vi "Result.Attributes plus Numeric into Results Table.vi"(6 "Meas":T1[](array[typedef]) {"Status" items=["LOG", "PASS", "FAIL", "ERROR"]}, 7 "File Data Objs":T3[](array[typedef]), 8 "Show Only Failures":bool, 9 "Filter":string, 10 "Attribute Data":T7[](array[typedef]) {"Status" items=["LOG", "PASS", "FAIL", "ERROR"]}, 11 "Numeric Data":T5[](array[typedef]) {"Status" items=["LOG", "PASS", "FAIL", "ERROR"]}) -> (1 "Failing":bool, 3 "Results Table":T4[](array[typedef]))   [LabVIEW 2024]
uses:
  Result.Attribute.ctl
  Result.Measurement and Attribute Item Status.ctl
  Result.Numeric.ctl
  Result.Limit Type.ctl
  Result.Results Table Record.ctl
  Reports/Report.Result FileDataObject.ctl
  Result.Measurement Item.ctl
  <vilib>/Utility/error.llb/Trim Whitespace One-Sided.vi
panel:
  in  "N/A Filler":string="n/a"
  in  "Precision (3)":i16=3
  # "Step                          Name                                             Value                      Units    LimType       LL           UL          Result        Code                     Description"
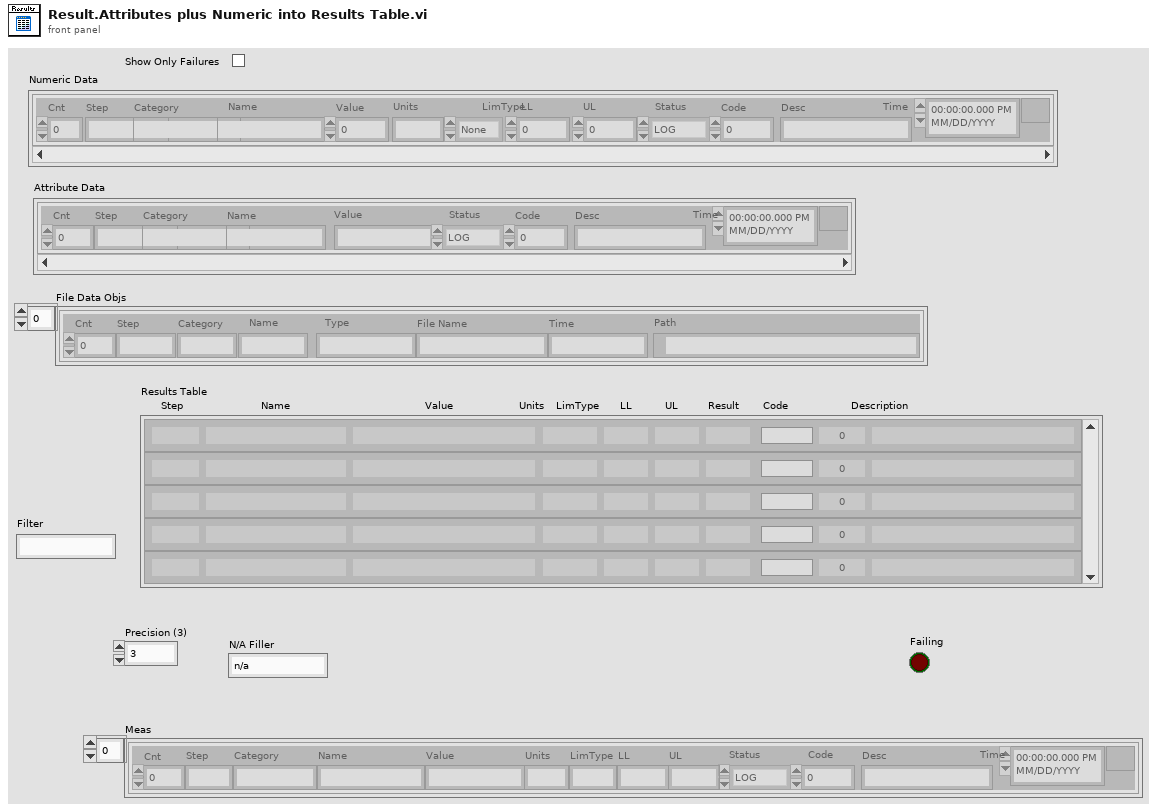
[diagram p1: front panel]
types:
  T1 = typedef "Result.Measurement Item.ctl" = cluster{"Cnt":i32, "Step":string, "Category":string, "Name":string, "Value":string, "Units":string, "LimType":string, "LL":string, "UL":string, "Status":T2, "Code":i32, "Desc":string, "Time":timestamp}
  T2 = typedef "Result.Measurement and Attribute Item Status.ctl" = i32
  T3 = typedef "Report.Result FileDataObject.ctl" = cluster{"Cnt":i32, "Step":string, "Category":string, "Name":string, "Type":string, "File Name":string, "Time":string, "Path":path}
  T4 = typedef "Result.Results Table Record.ctl" = cluster{"Cnt":i32, "Step":string, "Category":string, "Name":string, "Value":string, "Units":string, "LimType":string, "LL":string, "UL":string, "Status":string, "Status Color":u32, "Code":i32, "Desc":string}
  T5 = typedef "Result.Numeric.ctl" = cluster{"Cnt":i32, "Step":string, "Category":string, "Name":string, "Value":dbl, "Units":string, "LimType":T6, "LL":dbl, "UL":dbl, "Status":T2, "Code":i32, "Desc":string, "Time":timestamp}
  T6 = typedef "Result.Limit Type.ctl" = enum16{"None", "EQ", "NE", "GT", "LT", "GE", "LE", "GTLT", "GELE", "GELT", "GTLE", "LTGT", "LEGE", "LEGT", "LTGE", "Contains", "NotContains"}
  T7 = typedef "Result.Attribute.ctl" = cluster{"Cnt":i32, "Step":string, "Category":string, "Name":string, "Value":string, "Status":T2, "Code":i32, "Desc":string, "Time":timestamp}
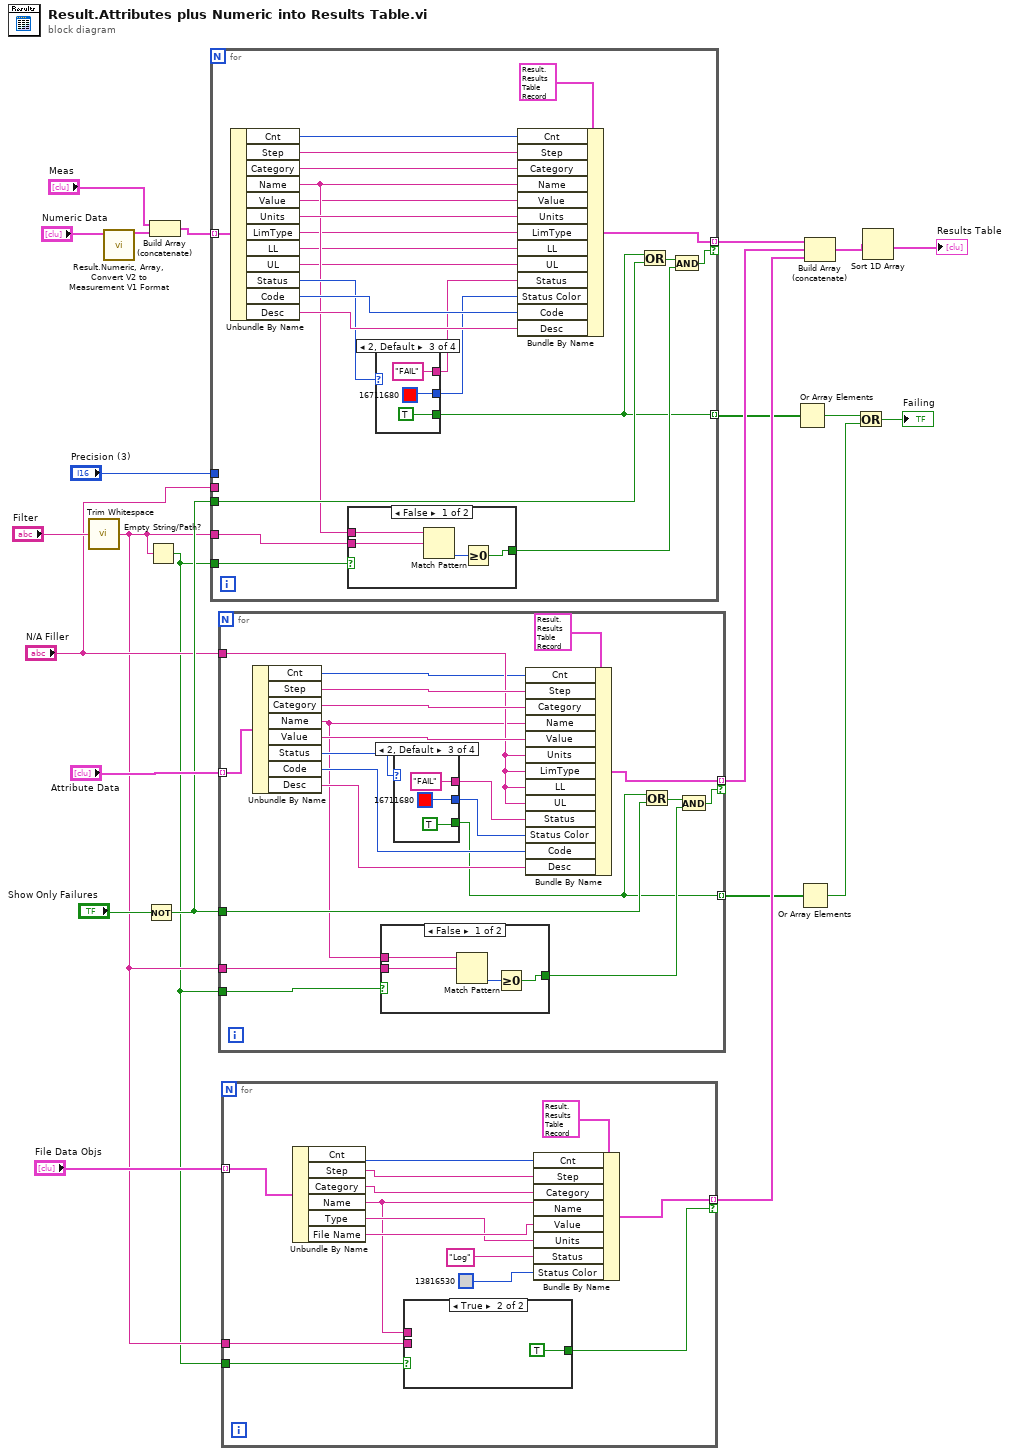
[diagram p0: block diagram]
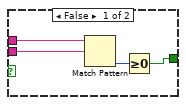
[diagram p2: hidden frame]
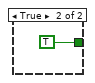
[diagram p3: hidden frame]
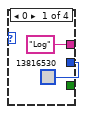
[diagram p4: hidden frame]
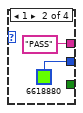
[diagram p5: hidden frame]
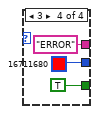
[diagram p6: hidden frame]
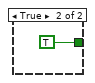
[diagram p7: hidden frame]
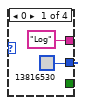
[diagram p8: hidden frame]
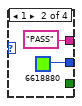
[diagram p9: hidden frame]
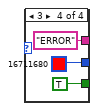
[diagram p10: hidden frame]
diagram:
  n1 = call <vilib>:"Trim Whitespace.vi"("string"="Filter") -> ("trimmed string"=w11:string)  [unwired: 1 in]
  n2 = call "Result.Numeric, Array, Convert V2 to Measurement V1 Format.vi"("Num In"="Numeric Data") -> ("Meas Out"=w8:T1[])  [unwired: 10 in]
  n3 = Not(x="Show Only Failures") -> (.not. x?=w16:bool)
  n4 = Empty String/Path?(string/path=w11) -> (empty?=w10:bool)
  n5 = Build Array (concatenate)("Meas", w8) -> (w6:T1[])
  n6 = for {
    tunnel: w6 -> [w46] mode=indexing
    tunnel: "Precision (3)" -> [_]
    tunnel: [w40] -> w22 mode=indexing if=w31
    tunnel: w16 -> [w35]
    tunnel: w11 -> [w33]
    tunnel: w10 -> [w29]
    tunnel: "N/A Filler" -> [_]
    tunnel: [w24] -> w5 mode=indexing
    n7 = Unbundle By Name(w46) -> ("Cnt"=w36:i32, "Step"=w45:string, "Category"=w44:string, "Name"=w34:string, "Value"=w28:string, "Units"=w41:string, "LimType"=w27:string, "LL"=w26:string, "UL"=w25:string, "Status"=w39:T2, "Code"=w42:i32, "Desc"=w43:string)
    n8 = case shown="False" w29 {
      tunnel: w33 -> [w51 _]
      tunnel: w34 -> [w50 _]
      tunnel: [w48 TRUE] -> w30
      frame False {
        n9 = Match Pattern(string=w50, regular expression=w51) -> (offset past match=w49:i32)  [unwired: 1 in, 3 out]
        n10 = Greater Or Equal To 0?(x=w49) -> (x >= 0?=w48:bool)
      }
      frame True {
      }
    }
    n11 = case shown="2, Default" w39 {
      tunnel: [u32 13816530 u32 6618880 u32 16711680 u32 16711680] -> w37
      tunnel: ["Log" "PASS" "FAIL" "ERROR"] -> w38
      tunnel: [_ _ TRUE TRUE] -> w24
      frame 0 {
      }
      frame 1 {
      }
      frame 2, Default {
      }
      frame 3 {
      }
    }
    n12 = Bundle By Name(cluster=T4 {"Cnt"=0, "Step"="", "Category"="", "Name"="", "Value"="", "Units"="", "LimType"="", "LL"="", "UL"="", "Status"="", "Status Color"=16448250, "Code"=0, "Desc"=""} ("Results Table Record"), "Cnt"=w36, "Step"=w45, "Category"=w44, "Name"=w34, "Value"=w28, "Units"=w41, "LimType"=w27, "LL"=w26, "UL"=w25, "Status"=w38, "Status Color"=w37, "Code"=w42, "Desc"=w43) -> (w40:T4)
    n13 = Or(x=w24, y=w35) -> (x .or. y?=w32:bool)
    n14 = And(x=w32, y=w30) -> (x .and. y?=w31:bool)
  }
  n15 = for {
    tunnel: "Attribute Data" -> [w82] mode=indexing
    tunnel: [w77] -> w21 mode=indexing if=w68
    tunnel: "N/A Filler" -> [w73]
    tunnel: w16 -> [w70]
    tunnel: w11 -> [w65]
    tunnel: w10 -> [w64]
    tunnel: [w63] -> w4 mode=indexing
    n16 = Unbundle By Name(w82) -> ("Cnt"=w71:i32, "Step"=w81:string, "Category"=w80:string, "Name"=w66:string, "Value"=w74:string, "Status"=w76:T2, "Code"=w78:i32, "Desc"=w79:string)
    n17 = case shown="False" w64 {
      tunnel: w65 -> [w87 _]
      tunnel: w66 -> [w86 _]
      tunnel: [w84 TRUE] -> w67
      frame False {
        n18 = Match Pattern(string=w86, regular expression=w87) -> (offset past match=w85:i32)  [unwired: 1 in, 3 out]
        n19 = Greater Or Equal To 0?(x=w85) -> (x >= 0?=w84:bool)
      }
      frame True {
      }
    }
    n20 = case shown="2, Default" w76 {
      tunnel: [u32 13816530 u32 6618880 u32 16711680 u32 16711680] -> w75
      tunnel: ["Log" "PASS" "FAIL" "ERROR"] -> w72
      tunnel: [_ _ TRUE TRUE] -> w63
      frame 0 {
      }
      frame 1 {
      }
      frame 2, Default {
      }
      frame 3 {
      }
    }
    n21 = Bundle By Name(cluster=T4 {"Cnt"=0, "Step"="", "Category"="", "Name"="", "Value"="", "Units"="", "LimType"="", "LL"="", "UL"="", "Status"="", "Status Color"=16448250, "Code"=0, "Desc"=""} ("Results Table Record"), "Cnt"=w71, "Step"=w81, "Category"=w80, "Name"=w66, "Value"=w74, "Units"=w73, "LimType"=w73, "LL"=w73, "UL"=w73, "Status"=w72, "Status Color"=w75, "Code"=w78, "Desc"=w79) -> (w77:T4)
    n22 = Or(x=w63, y=w70) -> (x .or. y?=w69:bool)
    n23 = And(x=w69, y=w67) -> (x .and. y?=w68:bool)
  }
  n24 = for {
    tunnel: "File Data Objs" -> [w111] mode=indexing
    tunnel: [w105] -> w12 mode=indexing if=w99
    tunnel: w11 -> [w103]
    tunnel: w10 -> [w102]
    n25 = Unbundle By Name(w111) -> ("Cnt"=w110:i32, "Step"=w109:string, "Category"=w108:string, "Name"=w104:string, "Type"=w106:string, "File Name"=w107:string)
    n26 = case shown="True" w102 {
      tunnel: w103 -> [w116 _]
      tunnel: w104 -> [w115 _]
      tunnel: [w113 TRUE] -> w99
      frame False {
        n27 = Match Pattern(string=w115, regular expression=w116) -> (offset past match=w114:i32)  [unwired: 1 in, 3 out]
        n28 = Greater Or Equal To 0?(x=w114) -> (x >= 0?=w113:bool)
      }
      frame True {
      }
    }
    n29 = Bundle By Name(cluster=T4 {"Cnt"=0, "Step"="", "Category"="", "Name"="", "Value"="", "Units"="", "LimType"="", "LL"="", "UL"="", "Status"="", "Status Color"=16448250, "Code"=0, "Desc"=""} ("Results Table Record"), "Cnt"=w110, "Step"=w109, "Category"=w108, "Name"=w104, "Value"=w107, "Units"=w106, "Status"="Log", "Status Color"=u32 13816530) -> (w105:T4)
  }
  n30 = Or Array Elements(Boolean array=w5) -> (logical OR=w3:bool)
  n31 = Or Array Elements(Boolean array=w4) -> (logical OR=w2:bool)
  n32 = Build Array (concatenate)(w22, w21, w12) -> (w19:T4[])
  n33 = Or(x=w3, y=w2) -> (x .or. y?=→"Failing":bool)
  n34 = Sort 1D Array(array=w19) -> (sorted array=→"Results Table":T4[])
